vi "NF WF1973_74 STAT Pres.vi"(8 "error in (no error)":errorcluster caption="Error IN", 11 "VISAsession":refnum<visa-resource-name>) -> (0 "error out":errorcluster caption="Error OUT", 3 "CopyVISAsession":refnum<visa-resource-name>)   [LabVIEW 2010]
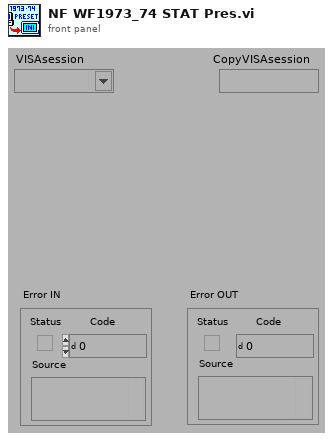
[diagram p1: front panel]
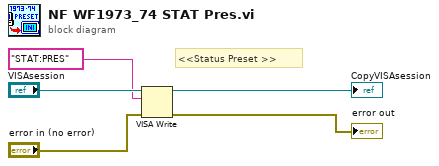
[diagram p0: block diagram]
diagram:
  # "<<Status Preset >>"
  n1 = VISA Write(VISA resource name="VISAsession", write buffer="STAT:PRES" ("文字列"), error in (no error)="error in (no error)") -> (VISA resource name out=→"CopyVISAsession":refnum<visa-resource-name>, error out=→"error out":errorcluster)  [unwired: 1 out]
